vi "GSI-HVSwitch2.ProcEvents.vi"(0 "i ref in":refnum<vi>, 5 "error in (no error)":errorcluster) -> (14 "i ref out":refnum<vi>, 19 "error out":errorcluster)   [LabVIEW 2014, in "GSI-HVSwitch2.lvlib"]
doc: "This method is used to define the events the object will listen to. Add your own events here."
uses:
  GSI-HVSwitch2.lvlib
  CSCore/BaseProcess/BaseProcess.event definition.ctl
  CSCore/CAEObj/CAEObj.event definition.ctl
  CSCore/BaseProcess/BaseProcess.descriptor string definition.ctl
  CSCore/BaseProcess/BaseProcess.lvlib
  CSCore/CAEObj/CAEObj.lvlib
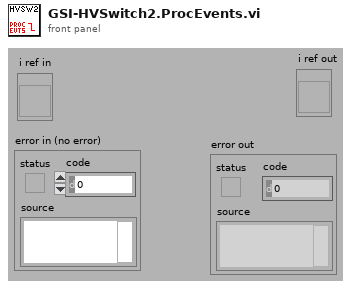
[diagram p1: front panel]
types:
  T1 = typedef "BaseProcess.lvlib/BaseProcess.event definition.ctl" = cluster{"CAEEvtDef":T2, "Data Descriptor":T3}
  T2 = typedef "CAEObj.lvlib/CAEObj.event definition.ctl" = cluster{"URL":string, "enable":bool, "ignoreResID":bool}
  T3 = typedef "BaseProcess.lvlib/BaseProcess.descriptor string definition.ctl" = string
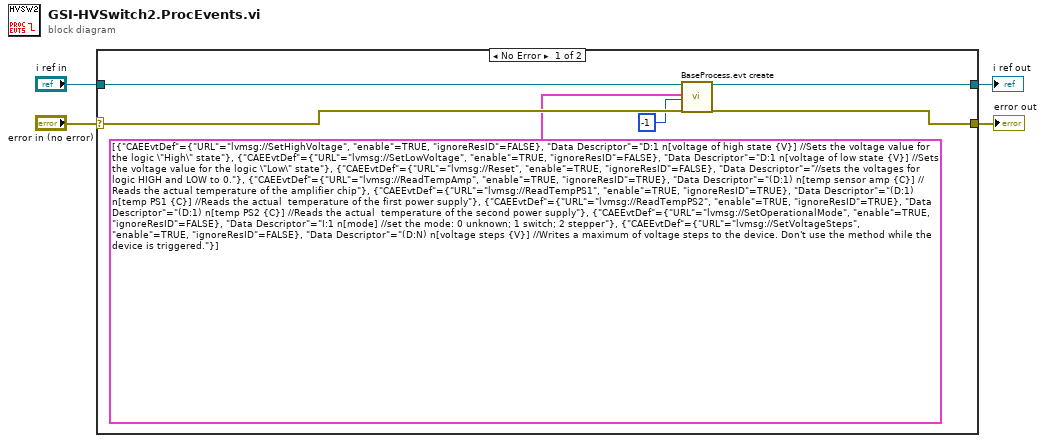
[diagram p0: block diagram]
diagram:
  n1 = case shown="No Error" "error in (no error)" {
    selector: "error in (no error)" -> [w9 w11]
    tunnel: "i ref in" -> [w10 w12]
    tunnel: [w5 w12] -> w3
    tunnel: [w6 w11] -> w2
    frame No Error {
      n2 = call "BaseProcess.evt create.vi"("i ref in"=w10, "newEvents"=T1[] [{"CAEEvtDef"={"URL"="lvmsg://SetHighVoltage", "enable"=TRUE, "ignoreResID"=FALSE}, "Data Descriptor"="D:1 n[voltage of high state {V}] //Sets the voltage value for the logic \"High\" state"}, {"CAEEvtDef"={"URL"="lvmsg://SetLowVoltage", "enable"=TRUE, "ignoreResID"=FALSE}, "Data Descriptor"="D:1 n[voltage of low state {V}] //Sets the voltage value for the logic \"Low\" state"}, {"CAEEvtDef"={"URL"="lvmsg://Reset", "enable"=TRUE, "ignoreResID"=FALSE}, "Data Descriptor"="//sets the voltages for logic HIGH and LOW to 0."}, {"CAEEvtDef"={"URL"="lvmsg://ReadTempAmp", "enable"=TRUE, "ignoreResID"=TRUE}, "Data Descriptor"="(D:1) n[temp sensor amp {C}] //Reads the actual temperature of the amplifier chip"}, {"CAEEvtDef"={"URL"="lvmsg://ReadTempPS1", "enable"=TRUE, "ignoreResID"=TRUE}, "Data Descriptor"="(D:1) n[temp PS1 {C}] //Reads the actual  temperature of the first power supply"}, {"CAEEvtDef"={"URL"="lvmsg://ReadTempPS2", "enable"=TRUE, "ignoreResID"=TRUE}, "Data Descriptor"="(D:1) n[temp PS2 {C}] //Reads the actual  temperature of the second power supply"}, {"CAEEvtDef"={"URL"="lvmsg://SetOperationalMode", "enable"=TRUE, "ignoreResID"=FALSE}, "Data Descriptor"="I:1 n[mode] //set the mode: 0 unknown; 1 switch; 2 stepper"}, {"CAEEvtDef"={"URL"="lvmsg://SetVoltageSteps", "enable"=TRUE, "ignoreResID"=FALSE}, "Data Descriptor"="(D:N) n[voltage steps {V}] //Writes a maximum of voltage steps to the device. Don't use the method while the device is triggered."}] ("new events"), "ms timeout (10000)"=-1, "error in (no error)"=w9) -> ("i ref out"=w5:refnum<vi>, "error out"=w6:errorcluster)  [unwired: 12 in, 2 out]
    }
    frame Error {
    }
  }
  "i ref out" <- w3
  "error out" <- w2
